vi "数据处理整合 (子VI).vi"(11 "枚举":enum16{"实时数据排序", "小时数据排序"}(ring)) -> (3 "已排序的数组":string[](array[string]))   [LabVIEW 2016, in "数据传输系统-05.lvlib"]
uses:
  <userlib>/_OpenG.lib/array/array.llb/Remove Duplicates from 1D Array (String)__ogtk.vi
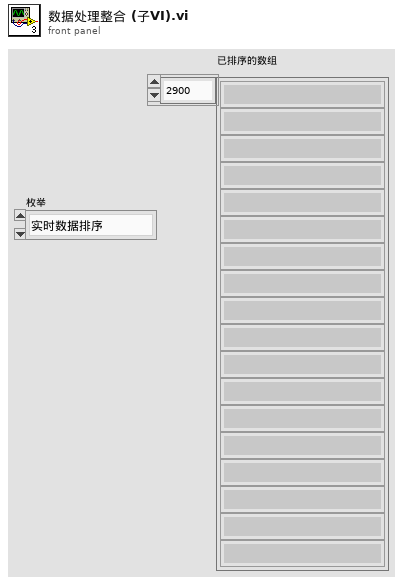
[diagram p1: front panel]
types:
  T1 = cluster{"PH":string[][], "CODCr":string[][], "氨氮":string[][], "CODMn":string[][], "总氮":string[][], "总磷":string[][], "电导率":string[][], "水温":string[][], "DO":string[][], "浊度":string[][], "叶绿素":string[][], "藻密度":string[][], "铜":string[][], "盐度":string[][], "水位":string[][], "流速":string[][], "瞬时流量":string[][], "累积流量":string[][], "亚硝酸盐":string[][], "硫化物":string[][], "ORP":string[][], "铅":string[][], "镉":string[][], "锌":string[][], "镍":string[][], "锰":string[][], "汞":string[][], "气温":string[][], "气压":string[][], "风速":string[][], "风向":string[][], "盐度 2":string[][], "磷酸盐":string[][], "硝氮":string[][], "氟化物":string[][], "挥发酚":string[][], "氯化物":string[][]}
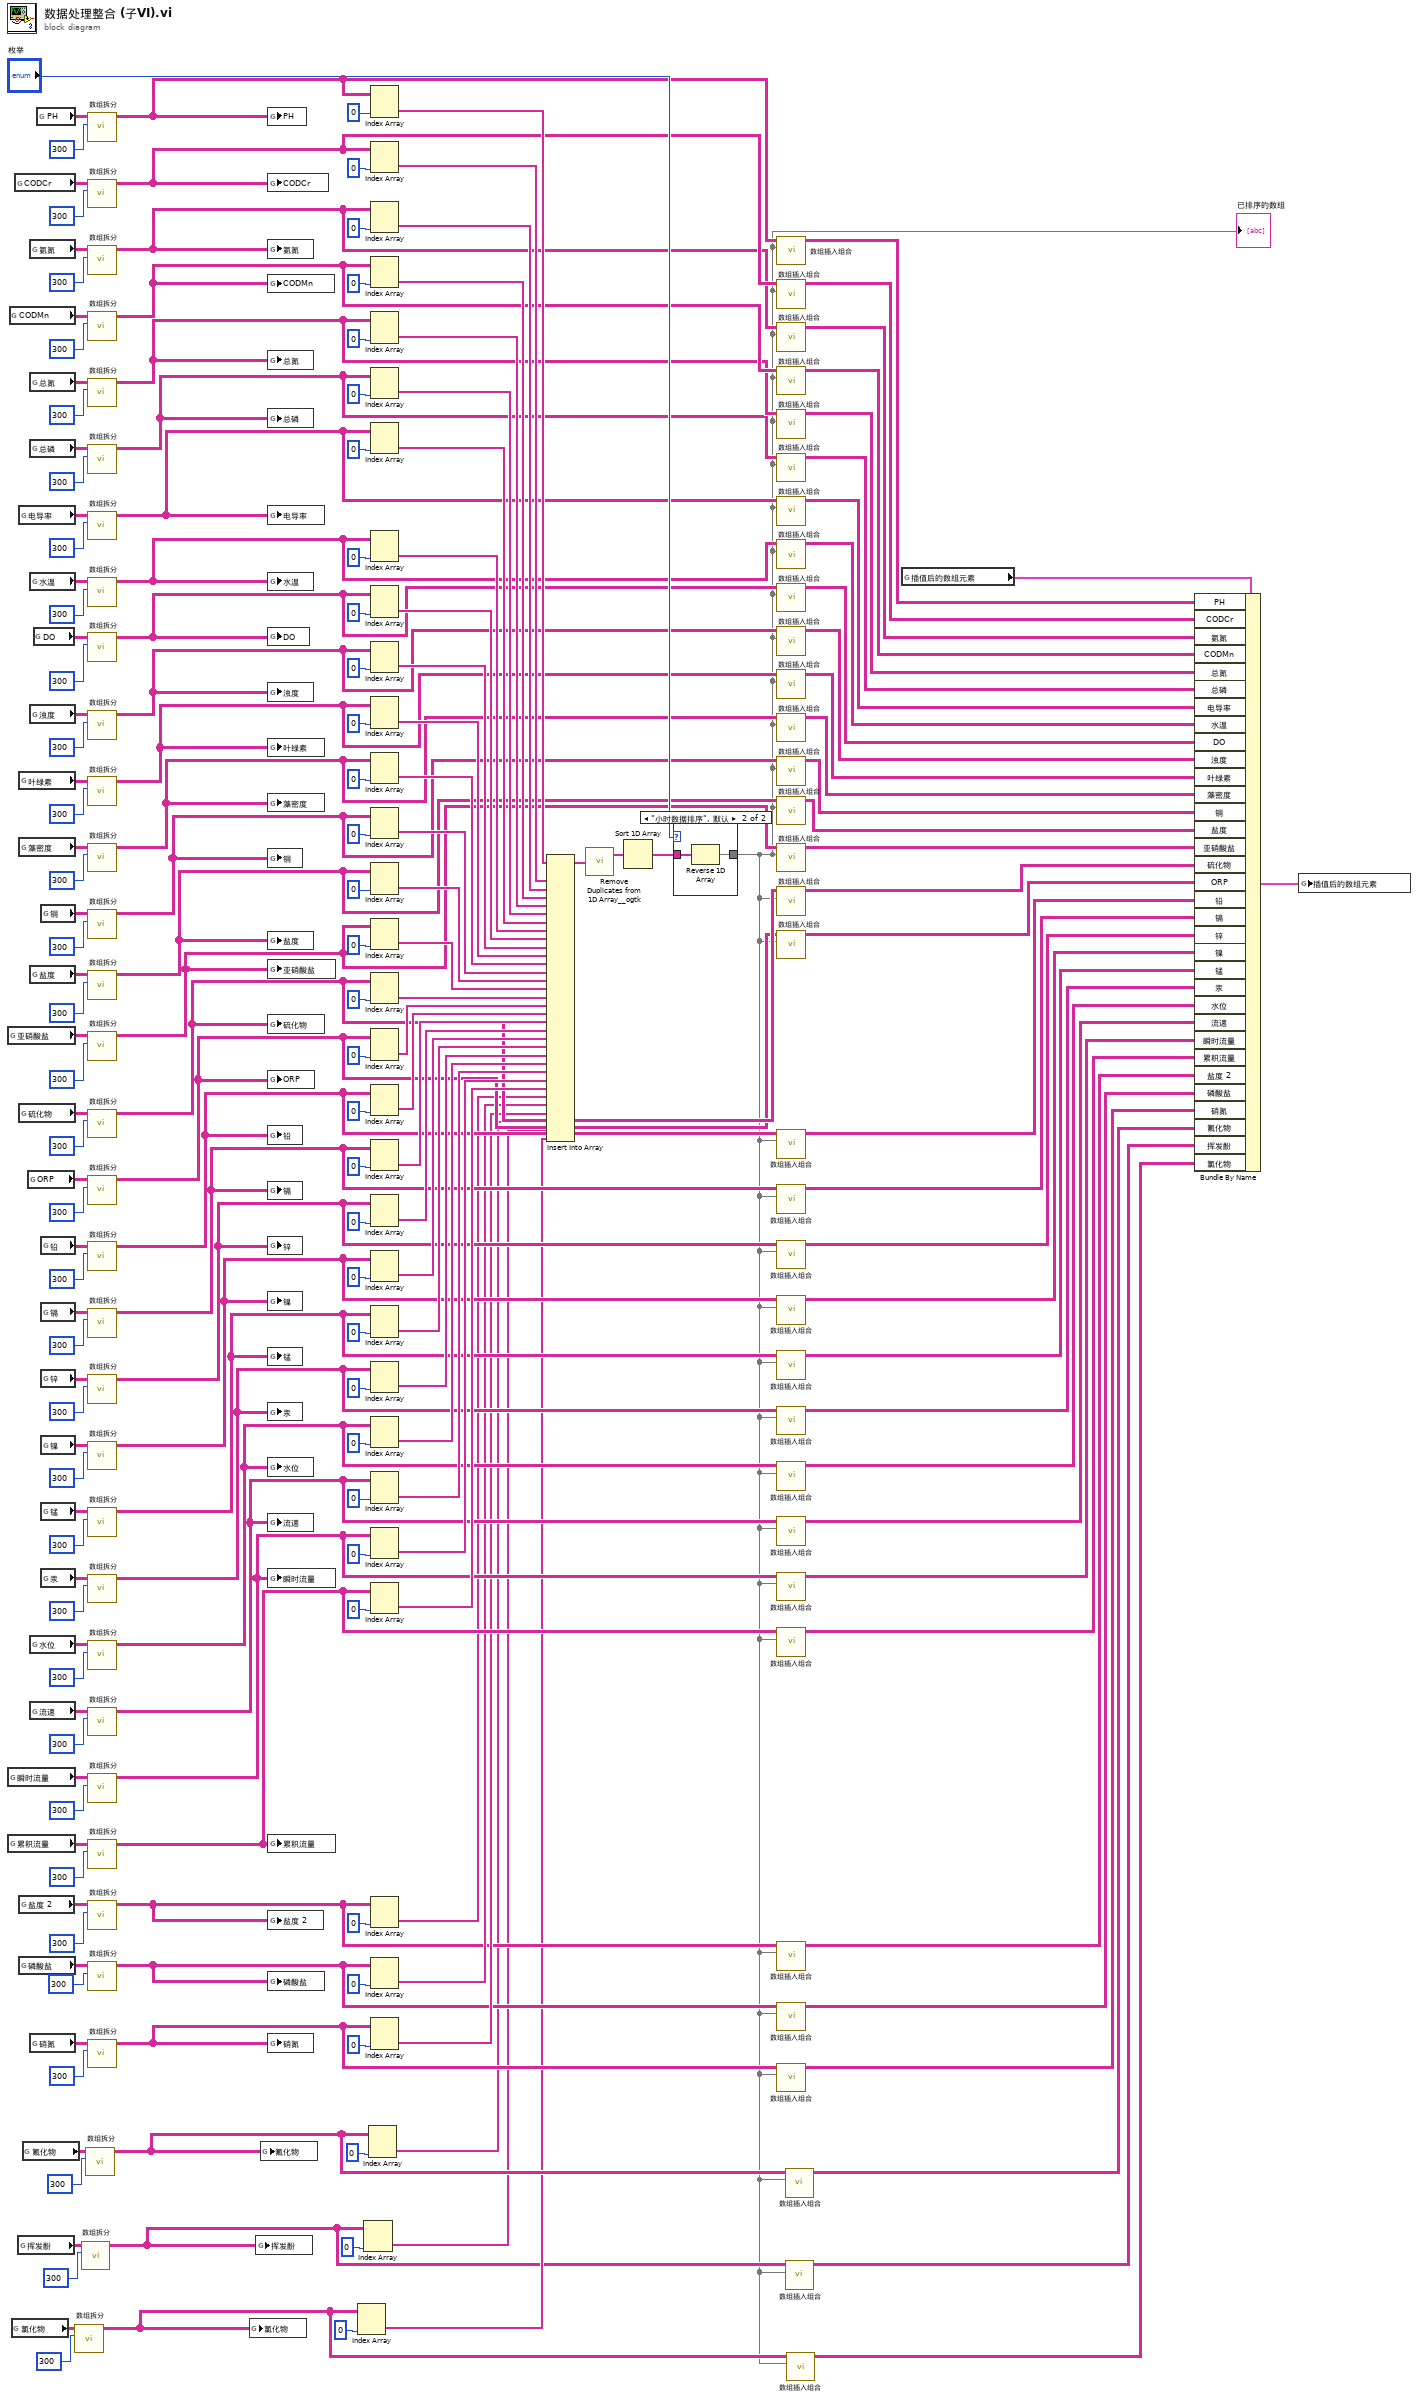
[diagram p0: block diagram]
diagram:
  n1 = global read "全局 所有参数.vi" "亚硝酸盐"() -> (w69:string[][])
  n2 = global read "全局 所有参数.vi" "瞬时流量"() -> (w45:string[][])
  n3 = global read "全局 所有参数.vi" "累积流量"() -> (w44:string[][])
  n4 = global read "全局 所有参数.vi" "CODMn"() -> (w108:string[][])
  n5 = global read "全局 所有参数.vi" "氯化物"() -> (w13:string[][])
  n6 = global read "全局 所有参数.vi" "CODCr"() -> (w114:string[][])
  n7 = global read "全局 所有参数.vi" "挥发酚"() -> (w14:string[][])
  n8 = global read "全局 所有参数.vi" "电导率"() -> (w98:string[][])
  n9 = global read "全局 所有参数.vi" "叶绿素"() -> (w85:string[][])
  n10 = global read "全局 所有参数.vi" "藻密度"() -> (w84:string[][])
  n11 = global read "全局 所有参数.vi" "硫化物"() -> (w68:string[][])
  n12 = global read "全局 所有参数.vi" "盐度 2"() -> (w31:string[][])
  n13 = global read "全局 所有参数.vi" "磷酸盐"() -> (w30:string[][])
  n14 = global read "全局 所有参数.vi" "氟化物"() -> (w19:string[][])
  n15 = global read "全局 所有参数.vi" "ORP"() -> (w67:string[][])
  n16 = global read "全局 所有参数.vi" "氨氮"() -> (w111:string[][])
  n17 = global read "全局 所有参数.vi" "总氮"() -> (w105:string[][])
  n18 = global read "全局 所有参数.vi" "总磷"() -> (w99:string[][])
  n19 = global read "全局 所有参数.vi" "水温"() -> (w97:string[][])
  n20 = global read "全局 所有参数.vi" "浊度"() -> (w86:string[][])
  n21 = global read "全局 所有参数.vi" "盐度"() -> (w82:string[][])
  n22 = global read "全局 所有参数.vi" "水位"() -> (w47:string[][])
  n23 = global read "全局 所有参数.vi" "流速"() -> (w46:string[][])
  n24 = global read "全局 所有参数.vi" "硝氮"() -> (w29:string[][])
  n25 = global read "全局 所有参数.vi" "DO"() -> (w96:string[][])
  n26 = global read "全局 所有参数.vi" "PH"() -> (w117:string[][])
  n27 = global read "全局 所有参数.vi" "铜"() -> (w83:string[][])
  n28 = global read "全局 所有参数.vi" "铅"() -> (w66:string[][])
  n29 = global read "全局 所有参数.vi" "镉"() -> (w65:string[][])
  n30 = global read "全局 所有参数.vi" "锌"() -> (w64:string[][])
  n31 = global read "全局 所有参数.vi" "镍"() -> (w63:string[][])
  n32 = global read "全局 所有参数.vi" "锰"() -> (w49:string[][])
  n33 = global read "全局 所有参数.vi" "汞"() -> (w48:string[][])
  n34 = call "数组拆分.vi"("拆分大小"=300, "输入数据"=w13) -> ("输出数组"=w5:string[][])  [unwired: 8 in, 1 out]
  n35 = call "数组拆分.vi"("拆分大小"=300, "输入数据"=w14) -> ("输出数组"=w6:string[][])  [unwired: 8 in, 1 out]
  n36 = call "数组拆分.vi"("拆分大小"=300, "输入数据"=w19) -> ("输出数组"=w9:string[][])  [unwired: 8 in, 1 out]
  n37 = call "数组拆分.vi"("拆分大小"=300, "输入数据"=w117) -> ("输出数组"=w116:string[][])  [unwired: 8 in, 1 out]
  n38 = call "数组拆分.vi"("拆分大小"=300, "输入数据"=w114) -> ("输出数组"=w113:string[][])  [unwired: 8 in, 1 out]
  n39 = call "数组拆分.vi"("拆分大小"=300, "输入数据"=w111) -> ("输出数组"=w110:string[][])  [unwired: 8 in, 1 out]
  n40 = call "数组拆分.vi"("拆分大小"=300, "输入数据"=w108) -> ("输出数组"=w107:string[][])  [unwired: 8 in, 1 out]
  n41 = call "数组拆分.vi"("拆分大小"=300, "输入数据"=w105) -> ("输出数组"=w104:string[][])  [unwired: 8 in, 1 out]
  n42 = call "数组拆分.vi"("拆分大小"=300, "输入数据"=w99) -> ("输出数组"=w92:string[][])  [unwired: 8 in, 1 out]
  n43 = call "数组拆分.vi"("拆分大小"=300, "输入数据"=w98) -> ("输出数组"=w93:string[][])  [unwired: 8 in, 1 out]
  n44 = call "数组拆分.vi"("拆分大小"=300, "输入数据"=w97) -> ("输出数组"=w94:string[][])  [unwired: 8 in, 1 out]
  n45 = call "数组拆分.vi"("拆分大小"=300, "输入数据"=w96) -> ("输出数组"=w95:string[][])  [unwired: 8 in, 1 out]
  n46 = call "数组拆分.vi"("拆分大小"=300, "输入数据"=w86) -> ("输出数组"=w81:string[][])  [unwired: 8 in, 1 out]
  n47 = call "数组拆分.vi"("拆分大小"=300, "输入数据"=w85) -> ("输出数组"=w77:string[][])  [unwired: 8 in, 1 out]
  n48 = call "数组拆分.vi"("拆分大小"=300, "输入数据"=w84) -> ("输出数组"=w78:string[][])  [unwired: 8 in, 1 out]
  n49 = call "数组拆分.vi"("拆分大小"=300, "输入数据"=w83) -> ("输出数组"=w79:string[][])  [unwired: 8 in, 1 out]
  n50 = call "数组拆分.vi"("拆分大小"=300, "输入数据"=w82) -> ("输出数组"=w80:string[][])  [unwired: 8 in, 1 out]
  n51 = call "数组拆分.vi"("拆分大小"=300, "输入数据"=w69) -> ("输出数组"=w62:string[][])  [unwired: 8 in, 1 out]
  n52 = call "数组拆分.vi"("拆分大小"=300, "输入数据"=w68) -> ("输出数组"=w61:string[][])  [unwired: 8 in, 1 out]
  n53 = call "数组拆分.vi"("拆分大小"=300, "输入数据"=w67) -> ("输出数组"=w60:string[][])  [unwired: 8 in, 1 out]
  n54 = call "数组拆分.vi"("拆分大小"=300, "输入数据"=w66) -> ("输出数组"=w59:string[][])  [unwired: 8 in, 1 out]
  n55 = call "数组拆分.vi"("拆分大小"=300, "输入数据"=w65) -> ("输出数组"=w58:string[][])  [unwired: 8 in, 1 out]
  n56 = call "数组拆分.vi"("拆分大小"=300, "输入数据"=w64) -> ("输出数组"=w57:string[][])  [unwired: 8 in, 1 out]
  n57 = call "数组拆分.vi"("拆分大小"=300, "输入数据"=w63) -> ("输出数组"=w56:string[][])  [unwired: 8 in, 1 out]
  n58 = call "数组拆分.vi"("拆分大小"=300, "输入数据"=w49) -> ("输出数组"=w43:string[][])  [unwired: 8 in, 1 out]
  n59 = call "数组拆分.vi"("拆分大小"=300, "输入数据"=w48) -> ("输出数组"=w41:string[][])  [unwired: 8 in, 1 out]
  n60 = call "数组拆分.vi"("拆分大小"=300, "输入数据"=w47) -> ("输出数组"=w42:string[][])  [unwired: 8 in, 1 out]
  n61 = call "数组拆分.vi"("拆分大小"=300, "输入数据"=w46) -> ("输出数组"=w40:string[][])  [unwired: 8 in, 1 out]
  n62 = call "数组拆分.vi"("拆分大小"=300, "输入数据"=w45) -> ("输出数组"=w39:string[][])  [unwired: 8 in, 1 out]
  n63 = call "数组拆分.vi"("拆分大小"=300, "输入数据"=w44) -> ("输出数组"=w38:string[][])  [unwired: 8 in, 1 out]
  n64 = call "数组拆分.vi"("拆分大小"=300, "输入数据"=w31) -> ("输出数组"=w25:string[][])  [unwired: 8 in, 1 out]
  n65 = call "数组拆分.vi"("拆分大小"=300, "输入数据"=w30) -> ("输出数组"=w24:string[][])  [unwired: 8 in, 1 out]
  n66 = call "数组拆分.vi"("拆分大小"=300, "输入数据"=w29) -> ("输出数组"=w23:string[][])  [unwired: 8 in, 1 out]
  n67 = global write "全局 所有参数.vi" "氯化物"(w5) -> ()
  n68 = global write "全局 所有参数.vi" "挥发酚"(w6) -> ()
  n69 = global write "全局 所有参数.vi" "氟化物"(w9) -> ()
  n70 = global write "全局 所有参数.vi" "PH"(w116) -> ()
  n71 = global write "全局 所有参数.vi" "CODCr"(w113) -> ()
  n72 = global write "全局 所有参数.vi" "氨氮"(w110) -> ()
  n73 = global write "全局 所有参数.vi" "CODMn"(w107) -> ()
  n74 = global write "全局 所有参数.vi" "总氮"(w104) -> ()
  n75 = global write "全局 所有参数.vi" "总磷"(w92) -> ()
  n76 = global write "全局 所有参数.vi" "电导率"(w93) -> ()
  n77 = global write "全局 所有参数.vi" "水温"(w94) -> ()
  n78 = global write "全局 所有参数.vi" "DO"(w95) -> ()
  n79 = global write "全局 所有参数.vi" "浊度"(w81) -> ()
  n80 = global write "全局 所有参数.vi" "叶绿素"(w77) -> ()
  n81 = global write "全局 所有参数.vi" "藻密度"(w78) -> ()
  n82 = global write "全局 所有参数.vi" "铜"(w79) -> ()
  n83 = global write "全局 所有参数.vi" "盐度"(w80) -> ()
  n84 = global write "全局 所有参数.vi" "亚硝酸盐"(w62) -> ()
  n85 = global write "全局 所有参数.vi" "硫化物"(w61) -> ()
  n86 = global write "全局 所有参数.vi" "ORP"(w60) -> ()
  n87 = global write "全局 所有参数.vi" "铅"(w59) -> ()
  n88 = global write "全局 所有参数.vi" "镉"(w58) -> ()
  n89 = global write "全局 所有参数.vi" "锌"(w57) -> ()
  n90 = global write "全局 所有参数.vi" "镍"(w56) -> ()
  n91 = global write "全局 所有参数.vi" "锰"(w43) -> ()
  n92 = global write "全局 所有参数.vi" "汞"(w41) -> ()
  n93 = global write "全局 所有参数.vi" "水位"(w42) -> ()
  n94 = global write "全局 所有参数.vi" "流速"(w40) -> ()
  n95 = global write "全局 所有参数.vi" "瞬时流量"(w39) -> ()
  n96 = global write "全局 所有参数.vi" "累积流量"(w38) -> ()
  n97 = global write "全局 所有参数.vi" "盐度 2"(w25) -> ()
  n98 = global write "全局 所有参数.vi" "磷酸盐"(w24) -> ()
  n99 = global write "全局 所有参数.vi" "硝氮"(w23) -> ()
  n100 = Index Array(array=w5, index (col)=0 ("索引 (行)")) -> (element=w7:string[])  [unwired: 1 in]
  n101 = Index Array(array=w6, index (col)=0 ("索引 (行)")) -> (element=w8:string[])  [unwired: 1 in]
  n102 = Index Array(array=w9, index (col)=0 ("索引 (行)")) -> (element=w10:string[])  [unwired: 1 in]
  n103 = Index Array(array=w116, index (col)=0 ("索引 (行)")) -> (element=w181:string[])  [unwired: 1 in]
  n104 = Index Array(array=w113, index (col)=0 ("索引 (行)")) -> (element=w182:string[])  [unwired: 1 in]
  n105 = Index Array(array=w110, index (col)=0 ("索引 (行)")) -> (element=w183:string[])  [unwired: 1 in]
  n106 = Index Array(array=w107, index (col)=0 ("索引 (行)")) -> (element=w184:string[])  [unwired: 1 in]
  n107 = Index Array(array=w104, index (col)=0 ("索引 (行)")) -> (element=w185:string[])  [unwired: 1 in]
  n108 = Index Array(array=w92, index (col)=0 ("索引 (行)")) -> (element=w186:string[])  [unwired: 1 in]
  n109 = Index Array(array=w93, index (col)=0 ("索引 (行)")) -> (element=w187:string[])  [unwired: 1 in]
  n110 = Index Array(array=w94, index (col)=0 ("索引 (行)")) -> (element=w188:string[])  [unwired: 1 in]
  n111 = Index Array(array=w95, index (col)=0 ("索引 (行)")) -> (element=w189:string[])  [unwired: 1 in]
  n112 = Index Array(array=w81, index (col)=0 ("索引 (行)")) -> (element=w190:string[])  [unwired: 1 in]
  n113 = Index Array(array=w77, index (col)=0 ("索引 (行)")) -> (element=w191:string[])  [unwired: 1 in]
  n114 = Index Array(array=w78, index (col)=0 ("索引 (行)")) -> (element=w192:string[])  [unwired: 1 in]
  n115 = Index Array(array=w79, index (col)=0 ("索引 (行)")) -> (element=w165:string[])  [unwired: 1 in]
  n116 = Index Array(array=w80, index (col)=0 ("索引 (行)")) -> (element=w164:string[])  [unwired: 1 in]
  n117 = Index Array(array=w62, index (col)=0 ("索引 (行)")) -> (element=w150:string[])  [unwired: 1 in]
  n118 = Index Array(array=w61, index (col)=0 ("索引 (行)")) -> (element=w151:string[])  [unwired: 1 in]
  n119 = Index Array(array=w60, index (col)=0 ("索引 (行)")) -> (element=w152:string[])  [unwired: 1 in]
  n120 = Index Array(array=w59, index (col)=0 ("索引 (行)")) -> (element=w142:string[])  [unwired: 1 in]
  n121 = Index Array(array=w58, index (col)=0 ("索引 (行)")) -> (element=w141:string[])  [unwired: 1 in]
  n122 = Index Array(array=w57, index (col)=0 ("索引 (行)")) -> (element=w140:string[])  [unwired: 1 in]
  n123 = Index Array(array=w56, index (col)=0 ("索引 (行)")) -> (element=w136:string[])  [unwired: 1 in]
  n124 = Index Array(array=w43, index (col)=0 ("索引 (行)")) -> (element=w135:string[])  [unwired: 1 in]
  n125 = Index Array(array=w41, index (col)=0 ("索引 (行)")) -> (element=w134:string[])  [unwired: 1 in]
  n126 = Index Array(array=w42, index (col)=0 ("索引 (行)")) -> (element=w126:string[])  [unwired: 1 in]
  n127 = Index Array(array=w40, index (col)=0 ("索引 (行)")) -> (element=w125:string[])  [unwired: 1 in]
  n128 = Index Array(array=w39, index (col)=0 ("索引 (行)")) -> (element=w124:string[])  [unwired: 1 in]
  n129 = Index Array(array=w38, index (col)=0 ("索引 (行)")) -> (element=w123:string[])  [unwired: 1 in]
  n130 = Index Array(array=w25, index (col)=0 ("索引 (行)")) -> (element=w28:string[])  [unwired: 1 in]
  n131 = Index Array(array=w24, index (col)=0 ("索引 (行)")) -> (element=w27:string[])  [unwired: 1 in]
  n132 = Index Array(array=w23, index (col)=0 ("索引 (行)")) -> (element=w26:string[])  [unwired: 1 in]
  n133 = Insert Into Array(array=w181, new element #1=w182, new element #2=w183, new element #3=w184, new element #4=w185, new element #5=w186, new element #6=w187, new element #7=w188, new element #8=w189, new element #9=w190, new element #10=w191, new element #11=w192, new element #12=w165, new element #13=w164, new element #14=w150, new element #15=w151, new element #16=w152, new element #17=w142, new element #18=w141, new element #19=w140, new element #20=w136, new element #21=w135, new element #22=w134, new element #23=w126, new element #24=w125, new element #25=w124, new element #26=w123, new element #27=w28, new element #28=w27, new element #29=w26, new element #30=w10, new element #31=w8, new element #32=w7) -> (w193:string[])  [unwired: 1 in]
  n134 = call-poly <userlib>:"Remove Duplicates from 1D Array__ogtk.vi"("Input Array"=w193) -> ("Output Array"=w180:string[])  [unwired: 1 out]
  n135 = Sort 1D Array(array=w180) -> (sorted array=w166:string[])
  n136 = case shown="\"小时数据排序\", 默认" "枚举" {
    tunnel: w166 -> [w206 w208]
    tunnel: [w206 w207] -> w4
    frame "实时数据排序" {
    }
    frame "小时数据排序", Default {
      n137 = Reverse 1D Array(array=w208) -> (reversed array=w207:string[])
    }
  }
  "已排序的数组" <- w4
  n138 = call "数组插入组合.vi"("排序后的一维数组"=w4, "输入数组"=w116) -> ("输出结果"=w194:string[][])  [unwired: 9 in]
  n139 = call "数组插入组合.vi"("排序后的一维数组"=w4, "输入数组"=w113) -> ("输出结果"=w195:string[][])  [unwired: 9 in]
  n140 = call "数组插入组合.vi"("排序后的一维数组"=w4, "输入数组"=w110) -> ("输出结果"=w196:string[][])  [unwired: 9 in]
  n141 = call "数组插入组合.vi"("排序后的一维数组"=w4, "输入数组"=w107) -> ("输出结果"=w197:string[][])  [unwired: 9 in]
  n142 = call "数组插入组合.vi"("排序后的一维数组"=w4, "输入数组"=w104) -> ("输出结果"=w198:string[][])  [unwired: 9 in]
  n143 = call "数组插入组合.vi"("排序后的一维数组"=w4, "输入数组"=w92) -> ("输出结果"=w199:string[][])  [unwired: 9 in]
  n144 = call "数组插入组合.vi"("排序后的一维数组"=w4, "输入数组"=w93) -> ("输出结果"=w200:string[][])  [unwired: 9 in]
  n145 = call "数组插入组合.vi"("排序后的一维数组"=w4, "输入数组"=w94) -> ("输出结果"=w201:string[][])  [unwired: 9 in]
  n146 = call "数组插入组合.vi"("排序后的一维数组"=w4, "输入数组"=w95) -> ("输出结果"=w202:string[][])  [unwired: 9 in]
  n147 = call "数组插入组合.vi"("排序后的一维数组"=w4, "输入数组"=w81) -> ("输出结果"=w203:string[][])  [unwired: 9 in]
  n148 = call "数组插入组合.vi"("排序后的一维数组"=w4, "输入数组"=w77) -> ("输出结果"=w204:string[][])  [unwired: 9 in]
  n149 = call "数组插入组合.vi"("排序后的一维数组"=w4, "输入数组"=w78) -> ("输出结果"=w205:string[][])  [unwired: 9 in]
  n150 = call "数组插入组合.vi"("排序后的一维数组"=w4, "输入数组"=w79) -> ("输出结果"=w163:string[][])  [unwired: 9 in]
  n151 = call "数组插入组合.vi"("排序后的一维数组"=w4, "输入数组"=w80) -> ("输出结果"=w162:string[][])  [unwired: 9 in]
  n152 = call "数组插入组合.vi"("排序后的一维数组"=w4, "输入数组"=w62) -> ("输出结果"=w155:string[][])  [unwired: 9 in]
  n153 = call "数组插入组合.vi"("排序后的一维数组"=w4, "输入数组"=w61) -> ("输出结果"=w153:string[][])  [unwired: 9 in]
  n154 = call "数组插入组合.vi"("排序后的一维数组"=w4, "输入数组"=w60) -> ("输出结果"=w154:string[][])  [unwired: 9 in]
  n155 = call "数组插入组合.vi"("排序后的一维数组"=w4, "输入数组"=w59) -> ("输出结果"=w145:string[][])  [unwired: 9 in]
  n156 = call "数组插入组合.vi"("排序后的一维数组"=w4, "输入数组"=w58) -> ("输出结果"=w144:string[][])  [unwired: 9 in]
  n157 = call "数组插入组合.vi"("排序后的一维数组"=w4, "输入数组"=w57) -> ("输出结果"=w143:string[][])  [unwired: 9 in]
  n158 = call "数组插入组合.vi"("排序后的一维数组"=w4, "输入数组"=w56) -> ("输出结果"=w133:string[][])  [unwired: 9 in]
  n159 = call "数组插入组合.vi"("排序后的一维数组"=w4, "输入数组"=w43) -> ("输出结果"=w132:string[][])  [unwired: 9 in]
  n160 = call "数组插入组合.vi"("排序后的一维数组"=w4, "输入数组"=w41) -> ("输出结果"=w131:string[][])  [unwired: 9 in]
  n161 = call "数组插入组合.vi"("排序后的一维数组"=w4, "输入数组"=w42) -> ("输出结果"=w122:string[][])  [unwired: 9 in]
  n162 = call "数组插入组合.vi"("排序后的一维数组"=w4, "输入数组"=w40) -> ("输出结果"=w121:string[][])  [unwired: 9 in]
  n163 = call "数组插入组合.vi"("排序后的一维数组"=w4, "输入数组"=w39) -> ("输出结果"=w120:string[][])  [unwired: 9 in]
  n164 = call "数组插入组合.vi"("排序后的一维数组"=w4, "输入数组"=w38) -> ("输出结果"=w119:string[][])  [unwired: 9 in]
  n165 = call "数组插入组合.vi"("排序后的一维数组"=w4, "输入数组"=w25) -> ("输出结果"=w22:string[][])  [unwired: 9 in]
  n166 = call "数组插入组合.vi"("排序后的一维数组"=w4, "输入数组"=w24) -> ("输出结果"=w21:string[][])  [unwired: 9 in]
  n167 = call "数组插入组合.vi"("排序后的一维数组"=w4, "输入数组"=w23) -> ("输出结果"=w20:string[][])  [unwired: 9 in]
  n168 = call "数组插入组合.vi"("排序后的一维数组"=w4, "输入数组"=w9) -> ("输出结果"=w3:string[][])  [unwired: 9 in]
  n169 = call "数组插入组合.vi"("排序后的一维数组"=w4, "输入数组"=w6) -> ("输出结果"=w2:string[][])  [unwired: 9 in]
  n170 = call "数组插入组合.vi"("排序后的一维数组"=w4, "输入数组"=w5) -> ("输出结果"=w1:string[][])  [unwired: 9 in]
  n171 = global read "插值后的新数组.vi" "插值后的数组元素"() -> (w159:T1)
  n172 = Bundle By Name(cluster=w159, "PH"=w194, "CODCr"=w195, "氨氮"=w196, "CODMn"=w197, "总氮"=w198, "总磷"=w199, "电导率"=w200, "水温"=w201, "DO"=w202, "浊度"=w203, "叶绿素"=w204, "藻密度"=w205, "铜"=w163, "盐度"=w162, "亚硝酸盐"=w155, "硫化物"=w153, "ORP"=w154, "铅"=w145, "镉"=w144, "锌"=w143, "镍"=w133, "锰"=w132, "汞"=w131, "水位"=w122, "流速"=w121, "瞬时流量"=w120, "累积流量"=w119, "盐度 2"=w22, "磷酸盐"=w21, "硝氮"=w20, "氟化物"=w3, "挥发酚"=w2, "氯化物"=w1) -> (w149:T1)
  n173 = global write "插值后的新数组.vi" "插值后的数组元素"(w149) -> ()
